vi "NI VeriStand - Close Multiple Waveforms Write Session (DBL).vi"(8 "error in (no error)":errorcluster, 11 "Multiple Waveforms Write Session (DBL)":refnum<class "Multiple Waveforms Write (DBL).lvclass">) -> (0 "error out":errorcluster)   [LabVIEW 2020, in "NI_VS Custom Device Waveform API.lvlib" / "Multiple Waveforms Write (DBL).lvclass"]
doc: "Closes a waveform read or write session. Wire data to the <B>Single Waveform Read Session (DBL)</B> input to specify the instance to use."
uses:
  Multiple Waveforms Write (DBL).lvclass
  D:/p4/penguin/lvaddon/Veristand/master/src/LabVIEW/vilib/NI VeriStand/Custom Device Waveform API/Waveform Session.lvclass
  Waveform Session.lvclass/Waveform Session.ctl
  Multiple Waveforms Write (DBL).lvclass/Multiple Waveforms Write (DBL).ctl
  Internal Comm Classes/WPL Comm/WPL Comm (2D DBL)/WPL Comm (2D DBL).lvclass/WPL Comm (2D DBL).ctl
  Internal Comm Classes/WPL Comm/WPL Comm.lvclass/WPL Comm.ctl
  Internal Comm Classes/WPL Comm/WPL Comm (2D DBL)/Set 2D DBL Q on Variant.vi
  Internal Comm Classes/WPL Comm/WPL_close waveform.vi
  Internal Comm Classes/WPL Comm/Convert Q Error to Shutdown Error.vi
  Internal Comm Classes/WPL Comm/Set ErrorQ on Variant.vi
  Internal Comm Classes/WPL Comm/Send WPL Command.vi
  Internal Comm Classes/WPL Comm/WPL Comm (2D DBL)/WPL Comm (2D DBL).lvclass
  D:/p4/penguin/lvaddon/Veristand/master/src/LabVIEW/vilib/NI VeriStand/Custom Device Waveform API/Internal Comm Classes/WPL Comm/WPL Comm.lvclass
  <vilib>/Utility/error.llb/Error Cluster From Error Code.vi
  Waveform Session.lvclass
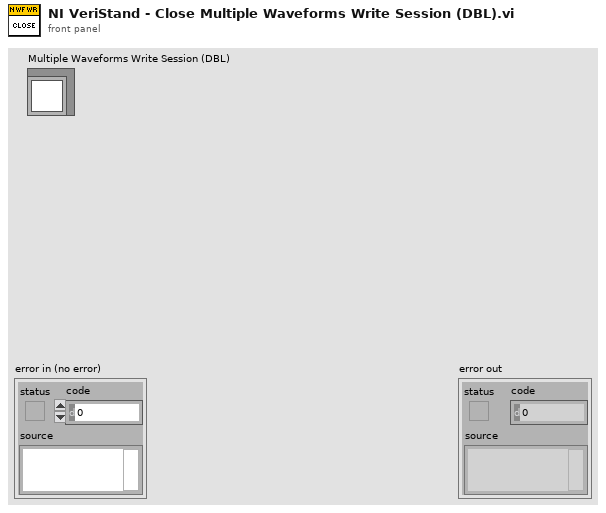
[diagram p1: front panel]
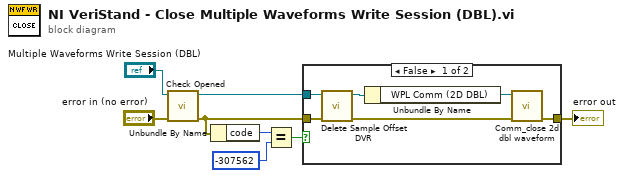
[diagram p0: block diagram]
diagram:
  n1 = call "Check Opened.vi"("error in (no error)"="error in (no error)", "Waveform Session in"="Multiple Waveforms Write Session (DBL)") -> ("error out"=w2:errorcluster, "Waveform Session out"=w7:refnum<class "Multiple Waveforms Write (DBL).lvclass">)  [unwired: 8 in]
  n2 = Unbundle By Name(w2) -> ("code"=w3:i32)
  n3 = Equal?(x=w3, y=-307562 ("error code (0)")) -> (x = y?=w1:bool)
  n4 = case shown="False" w1 {
    tunnel: w7 -> [w14 _]
    tunnel: w2 -> [w10 w15]
    tunnel: [w9 w15] -> w5
    frame False {
      n5 = call "Delete Sample Offset DVR.vi"("error in (no error)"=w10, "Waveform Session in"=w14) -> ("error out"=w11:errorcluster, "Waveform Session out"=w13:refnum<class "Multiple Waveforms Write (DBL).lvclass">)  [unwired: 8 in]
      n6 = Unbundle By Name(w13) -> ("WPL Comm (2D DBL)"=w12:refnum<class "WPL Comm (2D DBL).lvclass">)
      n7 = call "Comm_close 2d dbl waveform.vi"("error in (no error)"=w11, "WPL Comm (2D DBL) in"=w12) -> ("error out"=w9:errorcluster)  [unwired: 9 in]
    }
    frame True {
    }
  }
  "error out" <- w5
